vi "Initialize Rx HW Channels for RT.vi"(9 "Rx Channels In":T2[](array[typedef])=[{"channel #"=0, "channel handle"=0, "labels settings for RT"=[]}, {"channel #"=0, "channel handle"=0, "labels settings for RT"=[]}, {"channel #"=0, "channel handle"=0, "labels settings for RT"=[]}, {"channel #"=0, "channel handle"=0, "labels settings for RT"=[]}] {"labels settings for RT"."Label Timestamp Channel Data Reference" format="%.0x"; "labels settings for RT"."Word Initial Raw Value" format="%032.0f"; "labels settings for RT"."Label Disable/Trigger Channel Reference" format="%.0x"; "labels settings for RT"."parameter driver data"."Tx parameter refs" format="%.0x"; "labels settings for RT"."SDI" format="%02b"; "labels settings for RT"."label" format="%.0o"}) -> (3 "Rx Channels Out":T2[](array[typedef]) {"labels settings for RT"."Label Timestamp Channel Data Reference" format="%.0x"; "labels settings for RT"."Word Initial Raw Value" format="%032.0f"; "labels settings for RT"."Label Disable/Trigger Channel Reference" format="%.0x"; "labels settings for RT"."parameter driver data"."Tx parameter refs" format="%.0x"; "labels settings for RT"."SDI" format="%02b"; "labels settings for RT"."label" format="%.0o"}, 4 "map from identifiers to indexes":T1)   [LabVIEW 2020, in "AIM ARINC 429 Engine.lvlib" / "Custom Device.lvlib"]
uses:
  Custom Device.lvlib
  Shared/RT Label Settings.ctl
  Shared/Label.ctl
  Shared/RT Parameters.ctl
  Shared/Parameter Definition.ctl
  <vilib>/NI/NI VeriStand Encoding and Decoding/Encoding.ctl
  <vilib>/NI VeriStand/Custom Device API/Custom Device Item Ref.ctl
  Shared/Transfer Type.ctl
  <vilib>/NI VeriStand/Custom Device API/Data Reference.ctl
  Shared/Map of Identifiers to Indexes.ctl
  <vilib>/NI VeriStand/Custom Device API/Custom Device API.lvlib
  <vilib>/NI/NI VeriStand Encoding and Decoding/Encoding and Decoding.lvlib
  Shared/RT Hardware Channel Settings.ctl
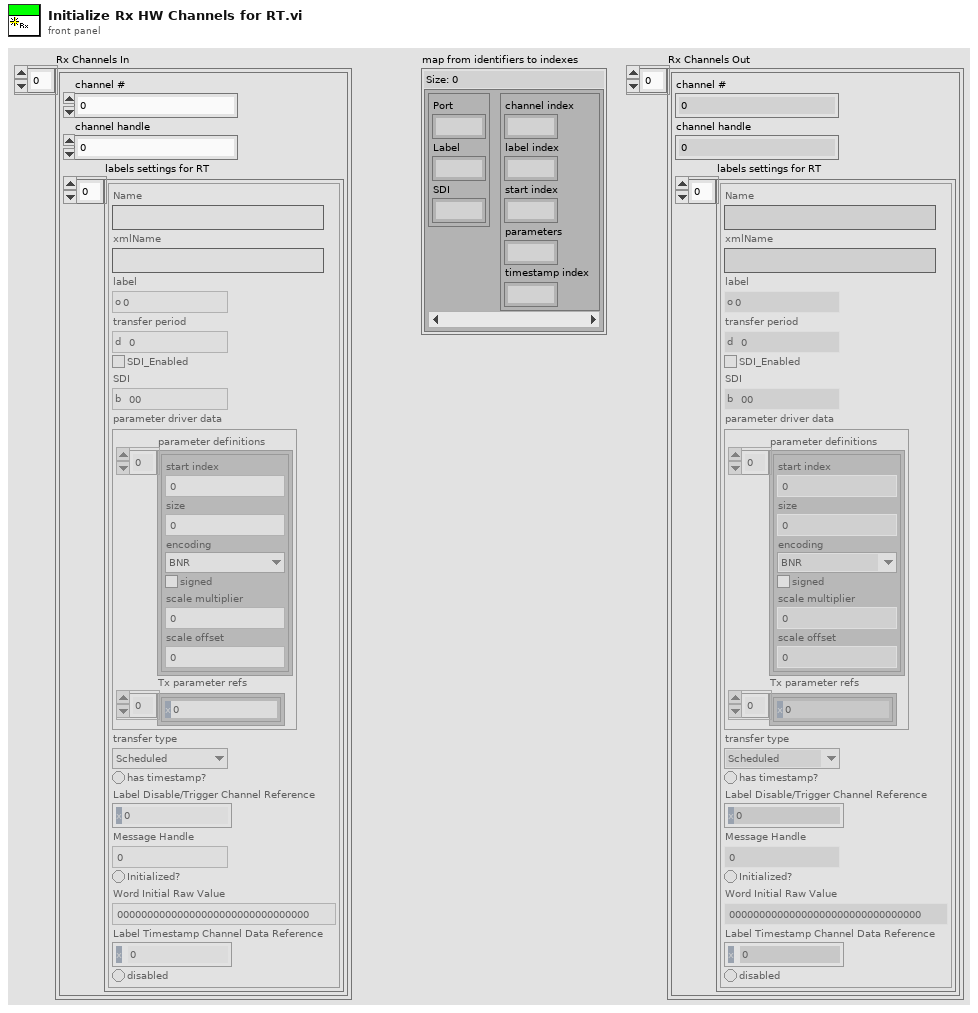
[diagram p1: front panel]
types:
  T1 = typedef "Map of Identifiers to Indexes.ctl" = map{cluster{"Port":u8, "Label":u8, "SDI":u8}, cluster{"channel index":i32, "label index":i32, "start index":i32, "parameters":i32, "timestamp index":i32}}
  T2 = typedef "RT Hardware Channel Settings.ctl" = cluster{"channel #":u16, "channel handle":u64, "labels settings for RT":T3[]}
  T3 = typedef "RT Label Settings.ctl" = cluster{"Name":string, "xmlName":string, "label":T4, "transfer period":u32, "SDI_Enabled":bool, "SDI":u8, "parameter driver data":T5, "transfer type":T9, "has timestamp?":bool, "Label Disable/Trigger Channel Reference":T8, "Message Handle":u64, "Initialized?":bool, "Word Initial Raw Value":u32, "Label Timestamp Channel Data Reference":T10, "disabled":bool}
  T4 = typedef "Label.ctl" = u8
  T5 = typedef "RT Parameters.ctl" = cluster{"parameter definitions":T6[], "Tx parameter refs":T8[]}
  T6 = typedef "Parameter Definition.ctl" = cluster{"start index":i32, "size":i32, "encoding":T7, "signed":bool, "scale multiplier":dbl, "scale offset":dbl}
  T7 = typedef "Encoding and Decoding.lvlib/Encoding.ctl" = enum16{"BNR", "BCD", "Discrete"}
  T8 = typedef "Custom Device API.lvlib/Custom Device Item Ref.ctl" = u64
  T9 = typedef "Transfer Type.ctl" = enum16{"Scheduled", "Acyclic", "Block", "Strobe"}
  T10 = typedef "Custom Device API.lvlib/Data Reference.ctl" = i32
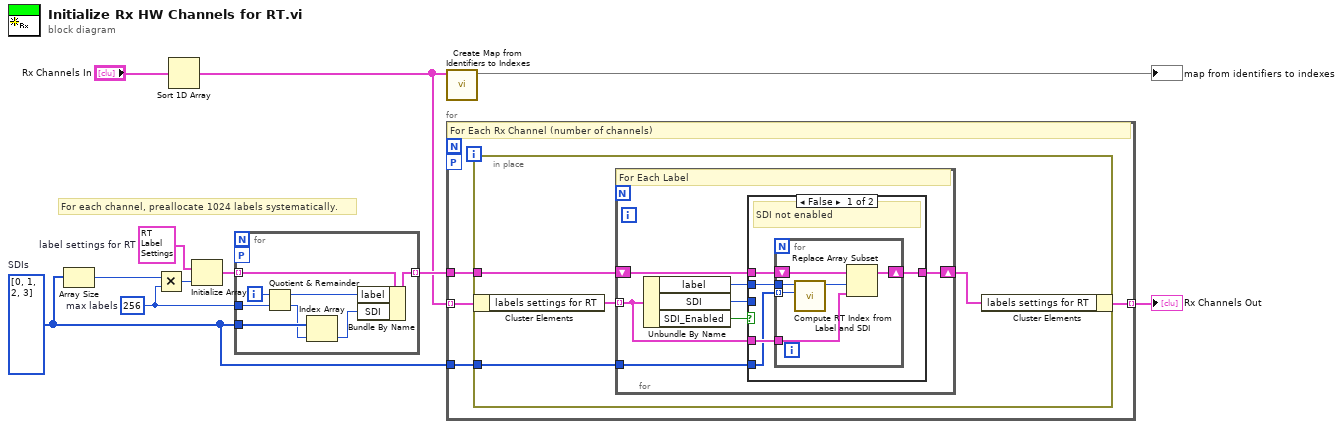
[diagram p0: block diagram]
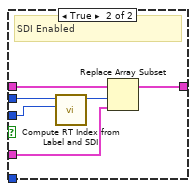
[diagram p2: hidden frame]
diagram:
  w5 = 256  # max labels
  w11 = T3 {"Name"="", "xmlName"="", "label"=0, "transfer period"=0, "SDI_Enabled"=FALSE, "SDI"=0, "parameter driver data"={"parameter definitions"=[], "Tx parameter refs"=[]}, "transfer type"=enum."Scheduled", "has timestamp?"=FALSE, "Label Disable/Trigger Channel Reference"=0, "Message Handle"=0, "Initialized?"=FALSE, "Word Initial Raw Value"=0, "Label Timestamp Channel Data Reference"=0, "disabled"=FALSE}  # label settings for RT
  w4 = u8[] [0, 1, 2, 3]  # SDIs
  # "For each channel, preallocate 1024 labels systematically."
  n1 = Array Size(array=w4) -> (size(s)=w8:i32)
  n2 = Multiply(x=w8, y=w5) -> (x*y=w10:i32)
  n3 = Sort 1D Array(array="Rx Channels In") -> (sorted array=w2:T2[])
  n4 = Initialize Array(w11, w10) -> (w9:T3[])
  n5 = for {
    tunnel: w9 -> [w17] mode=indexing
    tunnel: w5 -> [w18]
    tunnel: w4 -> [w16]
    tunnel: [w13] -> w7 mode=indexing
    workers-P: _ -> [_]
    i -> [w19]
    n6 = Quotient & Remainder(x=w19, y=w18) -> (x-y*floor(x/y)=w12:i32, floor(x/y)=w15:i32)
    n7 = Index Array(array=w16, index=w15) -> (element=w14:u8)
    n8 = Bundle By Name(cluster=w17, "label"=w12, "SDI"=w14) -> (w13:T3)
  }
  n9 = call "Create Map from Identifiers to Indexes.vi"("RT hardware channel data"=w2) -> ("map from identifiers to indexes"=→"map from identifiers to indexes":T1)  [unwired: 10 in]
  n10 = for {
    tunnel: w7 -> [w23]
    tunnel: w4 -> [w22]
    tunnel: w2 -> [w21] mode=indexing
    tunnel: [w20] -> w6 mode=indexing
    workers-P: _ -> [_]
    # "For Each Rx Channel (number of channels)"
    n11 = in-place {
      in-place-border: w23 -> [w27]
      in-place-border: w22 -> [w26]
      n12 = in-place-cluster #1(w21) -> ("labels settings for RT"=w25:T3[])
      n13 = for "Process each label" {
        tunnel: w25 -> [w32] mode=indexing
        shift-right: [w33] -> w24
        shift-left: w27 -> [w34]
        tunnel: w26 -> [w28]
        # "For Each Label"
        n14 = Unbundle By Name(w32) -> ("label"=w30:T4, "SDI"=w31:u8, "SDI_Enabled"=w29:bool)
        n15 = case shown="False" w29 {
          tunnel: w34 -> [w39 w51]
          tunnel: w32 -> [w36 w49]
          tunnel: w30 -> [w37 w48]
          tunnel: [w38 w50] -> w33
          tunnel: w31 -> [_ w47]
          tunnel: w28 -> [w35 _]
          frame False {
            # "SDI not enabled"
            n16 = for {
              tunnel: w37 -> [w41]
              tunnel: w36 -> [w43]
              shift-right: [w44] -> w38
              shift-left: w39 -> [w45]
              tunnel: w35 -> [w40] mode=indexing
              n17 = call "Compute RT Index from Label and SDI.vi"("SDI"=w40, "label"=w41) -> ("RT label index"=w42:i32)  [unwired: 9 in]
              n18 = Replace Array Subset(array=w45, new element=w43, index=w42) -> (w44:T3[])
            }
          }
          frame True {
            # "SDI Enabled"
            n19 = call "Compute RT Index from Label and SDI.vi"("SDI"=w47, "label"=w48) -> ("RT label index"=w46:i32)  [unwired: 9 in]
            n20 = Replace Array Subset(array=w51, new element=w49, index=w46) -> (w50:T3[])
          }
        }
      }
      n21 = in-place-cluster #1("labels settings for RT"=w24) -> (w20:T2)
    }
  }
  "Rx Channels Out" <- w6
